vi "Ctor.vi"(8 "error in (no error)":errorcluster, 10 "SQLite":refnum<class "SQLite.lvclass">) -> (0 "error out":errorcluster, 3 "User DB out":refnum<class "User DB.lvclass">)   [LabVIEW 2020, in "Summer of LabVIEW.lvlib" / "User DB.lvclass"]
uses:
  User DB.lvclass
  SQLite/SQLite.lvclass
  User DB.lvclass/User DB.ctl
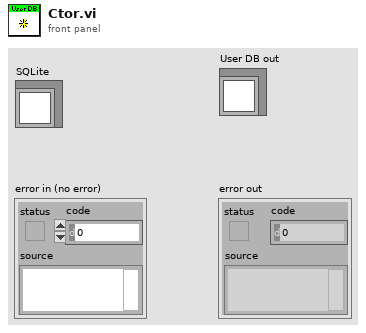
[diagram p1: front panel]
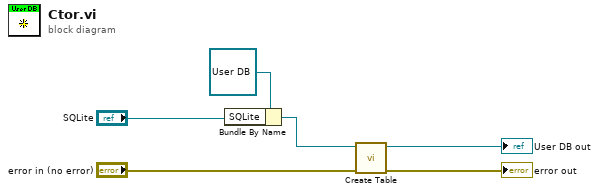
[diagram p0: block diagram]
diagram:
  n1 = Bundle By Name(cluster=refnum<class "User DB.lvclass"> refnum ("User DB in"), "SQLite"="SQLite") -> (w3:refnum<class "User DB.lvclass">)
  n2 = call "Create Table.vi"("error in (no error)"="error in (no error)", "User DB in"=w3) -> ("error out"=→"error out":errorcluster, "User DB out"=→"User DB out":refnum<class "User DB.lvclass">)  [unwired: 8 in]
